vi "Main.vi"() -> ()   [LabVIEW 2019]
panel:
  in  "LED":bool
  in  "stop":bool
  out "Y":dbl(graph)
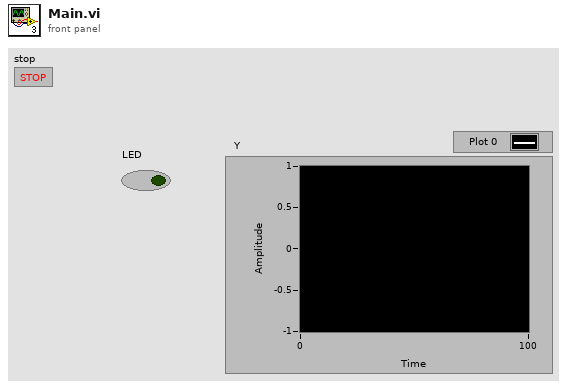
[diagram p1: front panel]
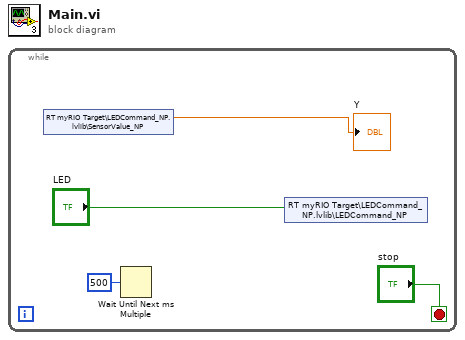
[diagram p0: block diagram]
diagram:
  n1 = while {
    stop <- "stop" stop-if-true
    n2 = shared-variable "RT myRIO Target\\LEDCommand_NP.lvlib\\SensorValue_NP"() -> (→"Y":dbl)  [unwired: 1 in, 1 out]
    n3 = Wait Until Next ms Multiple(millisecond multiple=u32 500) -> ()  [unwired: 1 out]
    n4 = shared-variable "RT myRIO Target\\LEDCommand_NP.lvlib\\LEDCommand_NP"("LED") -> ()  [unwired: 1 in, 1 out]
  }
